vi "sub_queue_algorithm.vi"() -> ()   [LabVIEW 2018]
uses:
  guess.ctl
panel:
  in  "solver (in)":cluster{"solved":bool, "values":string[]}[][](array[cluster]) caption="solver array"
  in  "queues":T1
  in  "operations":enum16{"next guess", "undo previous guess"}(ring)
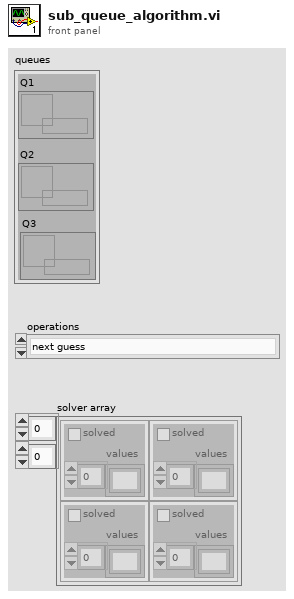
[diagram p1: front panel]
types:
  T1 = cluster{"Q1":refnum<queue>, "Q2":refnum<queue>, "Q3":refnum<queue>}
  T2 = typedef "guess.ctl" = cluster{"cell position":cluster{"row":i32, "col":i32}, "guess":string}
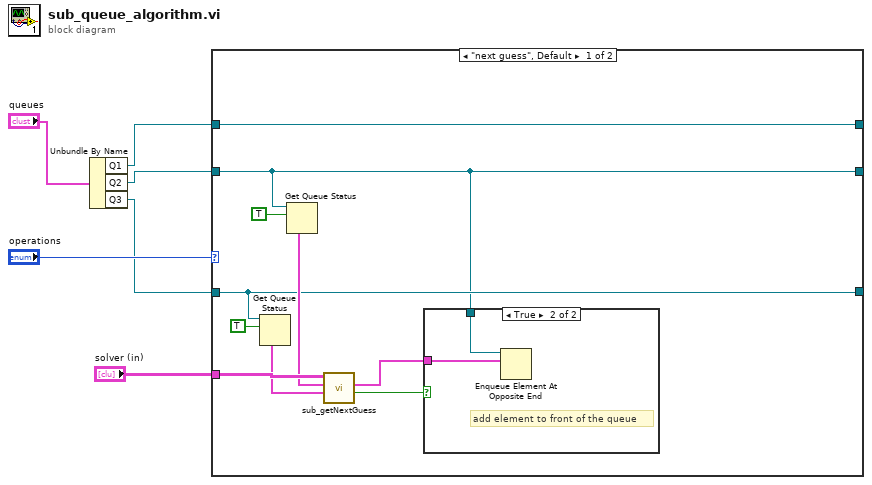
[diagram p0: block diagram]
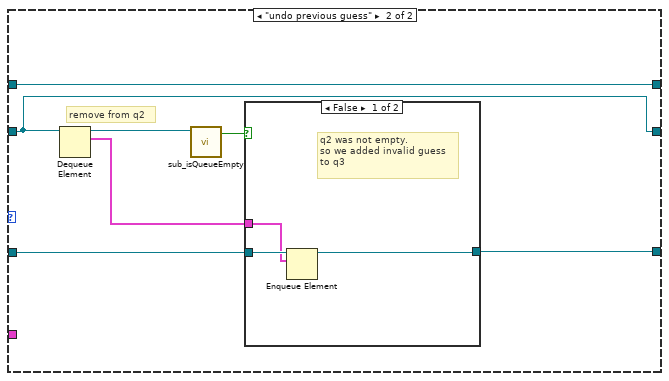
[diagram p3: hidden frame]
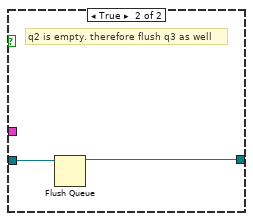
[diagram p4: hidden frame]
diagram:
  n1 = Unbundle By Name("queues") -> ("Q1"=w4:refnum<queue>, "Q2"=w3:refnum<queue>, "Q3"=w2:refnum<queue>)
  n2 = case shown="\"next guess\", Default" "operations" {
    tunnel: w3 -> [w8 w25]
    tunnel: w2 -> [w12 w24]
    tunnel: [w12 w22] -> _
    tunnel: [w8 w25] -> _
    tunnel: w4 -> [w16 w21]
    tunnel: [w16 w21] -> _
    tunnel: "solver (in)" -> [w15 _]
    frame "next guess", Default {
      n3 = Get Queue Status(queue=w12, return elements? (F)=TRUE) -> (elements=w10:T2[])  [unwired: 1 in, 7 out]
      n4 = Get Queue Status(queue=w8, return elements? (F)=TRUE) -> (elements=w13:T2[])  [unwired: 1 in, 7 out]
      n5 = call "sub_getNextGuess.vi"("invalid guesses"=w10, "current guess queue"=w13, "solver array"=w15) -> ("no valid guess ?"=w9:bool, "next guess"=w7:T2)  [unwired: 7 in]
      n6 = case shown="True" w9 {
        tunnel: w8 -> [_ w18]
        tunnel: w7 -> [_ w17]
        frame False {
        }
        frame True {
          # "add element to front of the queue"
          n7 = Enqueue Element At Opposite End(queue=w18, element=w17) -> ()  [unwired: 2 in, 3 out]
        }
      }
    }
    frame "undo previous guess" {
      # "remove from q2"
      n8 = Dequeue Element(queue=w25) -> (queue out=w20:refnum<queue>, element=w23:T2)  [unwired: 2 in, 2 out]
      n9 = call "sub_isQueueEmpty"("Q1"=w20) -> ("empty ?"=w19:bool)  [unwired: 10 in]
      n10 = case shown="False" w19 {
        tunnel: w24 -> [w28 w30]
        tunnel: w23 -> [w27 _]
        tunnel: [w26 w29] -> w22
        frame False {
          # "q2 was not empty. \nso we added invalid guess\nto q3"
          n11 = Enqueue Element(queue=w28, element=w27) -> (queue out=w26:refnum<queue>)  [unwired: 2 in, 2 out]
        }
        frame True {
          # "q2 is empty. therefore flush q3 as well"
          n12 = Flush Queue(queue=w30) -> (queue out=w29:refnum<queue>)  [unwired: 1 in, 2 out]
        }
      }
    }
  }
